vi "Pre Launch Init.vi"(11 "Client Controller in":refnum<class "Client Controller.lvclass">) -> (0 "error out":errorcluster, 3 "Client Controller out":refnum<class "Client Controller.lvclass">)   [LabVIEW 2017, in "Client Controller.lvlib" / "Client Controller.lvclass"]
doc: "(<B>Filename</B>: Actor Framework.lvlib:Actor.lvclass:Pre Launch Init.vi)\n\nDefines behavior that occurs after the Launch Actor method is invoked but before the actor's Actor Core method begins running.\n\nThe Pre Launch Init method is guaranteed to finish before the Launch Actor method returns to its caller and before the actor itself receives any messages. Any references that the Pre Launch Init method obtains are guaranteed to have the same lifetime as the actor itself. Any errors that the Pre Launch Init method returns will abort the launch.\n\nBy default, this method does nothing. A descendant class may override it to define behavior."
uses:
  Client Controller.lvclass
  MAL-Framework/user.lib/Common Components/Controller/Controller.lvclass
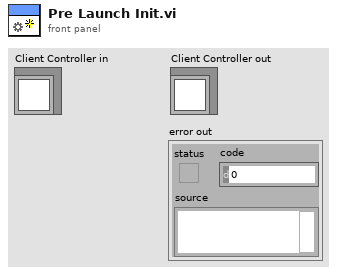
[diagram p1: front panel]
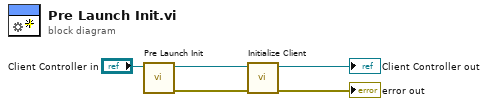
[diagram p0: block diagram]
diagram:
  n1 = call-parent "Pre Launch Init.vi"("Controller in"="Client Controller in") -> ("error out"=w1:errorcluster, "Controller out"=w4:refnum<class "Client Controller.lvclass">)  [unwired: 9 in]
  n2 = call-dynamic "Initialize Client.vi"("error in (no error)"=w1, "Client Controller in"=w4) -> ("error out"=→"error out":errorcluster, "Client Controller out"=→"Client Controller out":refnum<class "Client Controller.lvclass">)  [unwired: 8 in]
